vi "Power Supply Close Chain.vi"(5 "Power Supply Chain VISA Session":refnum<visa-resource-name>, 11 "error in (no error)":errorcluster) -> (15 "error out":errorcluster)   [LabVIEW 2017, in "Power Supply.lvclass"]
uses:
  Power Supply.lvclass
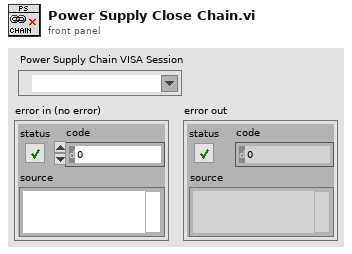
[diagram p1: front panel]
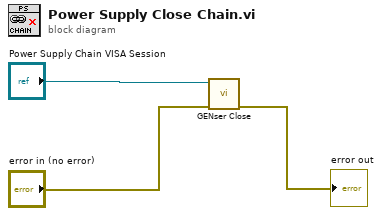
[diagram p0: block diagram]
diagram:
  n1 = call <instrlib>:"GENser Close.vi"("error"="error in (no error)", "VISA name"="Power Supply Chain VISA Session") -> ("error out"=→"error out":errorcluster)  [unwired: 9 in]
